vi "Read Multiple AIN.vi"() -> (0 "error out":errorcluster)   [LabVIEW 2020]
panel:
  out "Values":dbl[](array[numeric]) format="%.6f"
  in  "Channels":string[](array[string])=["AIN0", "AIN1", "AIN2", "AIN3"]
  in  "Config Values":dbl[](array[numeric])=[10.0, 0.0, 0.0] format="%.2f"
  out "Error String":string
  out "ConnectionType Out":i32
  out "DeviceType Out":i32
  in  "Identifier":string="LJM_idANY"
  in  "ConnectionType":string="LJM_ctANY"
  in  "DeviceType":string="LJM_dtANY"
  in  "Config Names":string[](array[string])=["AIN_ALL_RANGE", "AIN_ALL_RESOLUTION_INDEX", "AIN_ALL_SETTLING_US"]
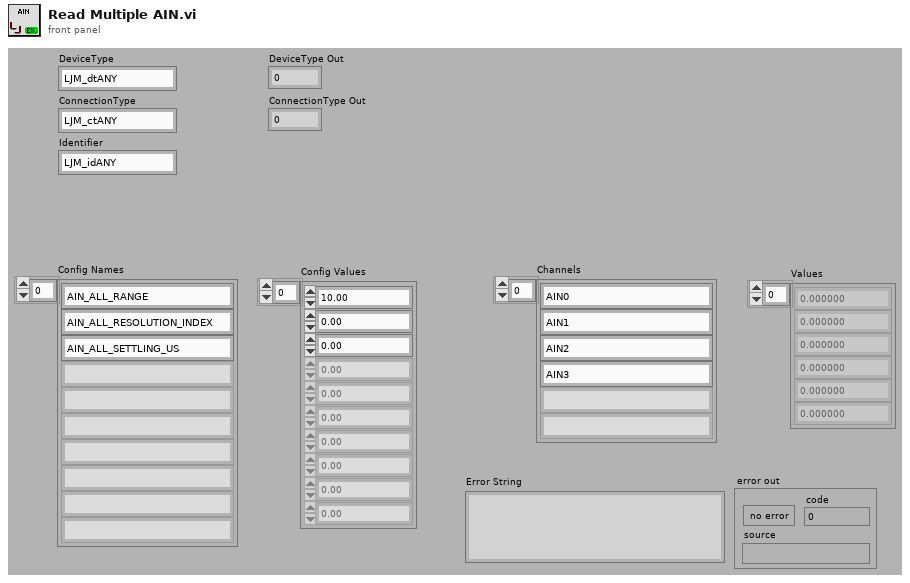
[diagram p1: front panel]
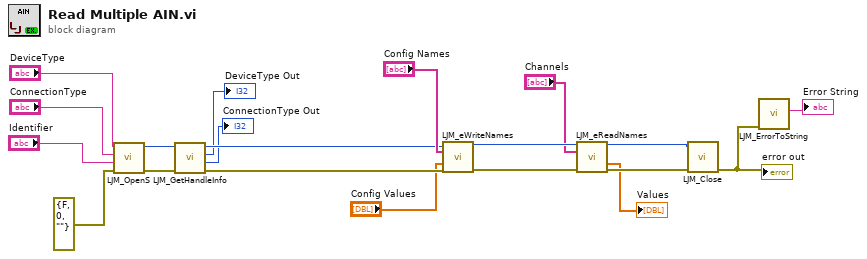
[diagram p0: block diagram]
diagram:
  n1 = call "LJM_OpenS.vi"("error in"=errorcluster {"status"=FALSE, "code"=0, "source"=""} ("error in (no error)"), "Identifier"="Identifier", "ConnectionType"="ConnectionType", "DeviceType"="DeviceType") -> ("error out"=w18:errorcluster, "Handle"=w16:i32)  [unwired: 6 in]
  n2 = call "LJM_GetHandleInfo.vi"("error in"=w18, "Handle In"=w16) -> ("error out"=w17:errorcluster, "ConnectionType"=→"ConnectionType Out":i32, "DeviceType"=→"DeviceType Out":i32, "Handle Out"=w15:i32)  [unwired: 2 in, 4 out]
  n3 = call "LJM_eWriteNames.vi"("Handle In"=w15, "aNames"="Config Names", "aValuesIn"="Config Values", "error in"=w17) -> ("Handle Out"=w5:i32, "error out"=w6:errorcluster)  [unwired: 9 in, 1 out]
  n4 = call "LJM_eReadNames.vi"("Handle In"=w5, "aNames"="Channels", "error in"=w6) -> ("Handle Out"=w3:i32, "aValuesOut"=→"Values":dbl[], "error out"=w4:errorcluster)  [unwired: 9 in, 1 out]
  n5 = call "LJM_Close.vi"("error in"=w4, "Handle"=w3) -> ("error out"=w9:errorcluster)  [unwired: 9 in]
  "error out" <- w9
  n6 = call "LJM_ErrorToString.vi"("error in"=w9) -> ("String"=→"Error String":string)  [unwired: 10 in]
